vi "LJUD_eDO.vi"(8 "error in":errorcluster, 9 "State":i32, 10 "Channel":i32, 11 "Handle In":i32) -> (0 "error out":errorcluster, 3 "Handle Out":i32)   [LabVIEW 2020]
doc: "This is an easy function to set the\nstate of a single digital output. The\ndirection of the DIO is automatically\nset to output.\n\nSee Sections 4.2 and 4.3 of the device's\ndatasheet for more information."
uses:
  labjackud.dll
panel:
  # "This is an easy function to set the\nstate of a single digital output.  The\ndirection of the DIO is automatically\nset to output.\n\nSee Sections 4.2 and 4.3 of the device's\ndatasheet for more information."
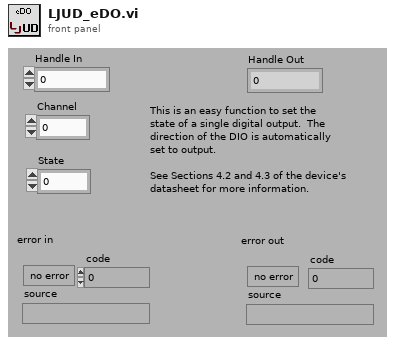
[diagram p1: front panel]
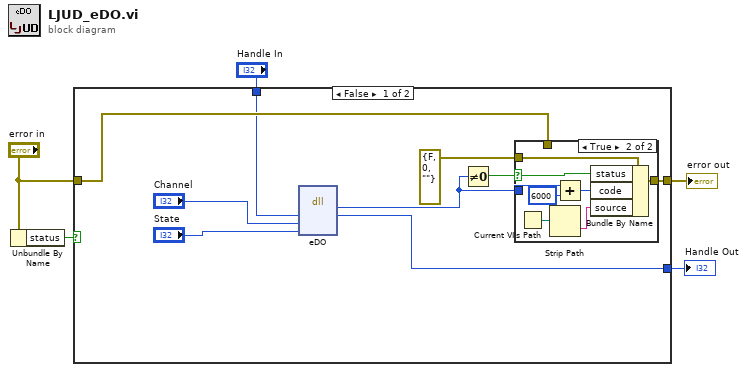
[diagram p0: block diagram]
diagram:
  n1 = Unbundle By Name("error in") -> ("status"=w4:bool)
  n2 = case shown="False" w4 {
    tunnel: [w11 w25] -> w5
    tunnel: "error in" -> [w10 w25]
    tunnel: "Handle In" -> [w7 w24]
    tunnel: [w6 w24] -> w1
    frame False {
      n3 = dll-call lib="labjackud.dll" fn="eDO"("Handle"=w7, "Channel"="Channel", "State"="State") -> (w12:i32, "Handle"=w6:i32)  [unwired: 5 in, 2 out]
      n4 = Not Equal To 0?(x=w12) -> (x != 0?=w13:bool)
      n5 = case shown="True" w13 {
        selector: w13 -> [_ w22]
        tunnel: [w15 w23] -> w11
        tunnel: errorcluster {"status"=FALSE, "code"=0, "source"=""} ("error IO") -> [_ w21]
        tunnel: w12 -> [_ w17]
        tunnel: w10 -> [w15 _]
        frame False {
        }
        frame True {
          n6 = Current VI's Path() -> (path=w19:path)
          n7 = Strip Path(path=w19) -> (name=w20:string)  [unwired: 1 out]
          n8 = Add(x=w17, y=6000) -> (x+y=w18:i32)
          n9 = Bundle By Name(cluster=w21, "status"=w22, "code"=w18, "source"=w20) -> (w23:errorcluster)
        }
      }
    }
    frame True {
    }
  }
  "error out" <- w5
  "Handle Out" <- w1
